vi "frequency measurement(2 notes).vi"() -> (0 "second note":dbl, 3 "first note":dbl)   [LabVIEW 2016]
uses:
  <vilib>/myRIO/Instrument Drivers/Onboard IO/AudioIn Block/typedefs/AudioIn Block Reference.ctl
  <vilib>/myRIO/Common/Instrument Driver Framework/Utilities/typedefs/myRIO Generic Hardware Reference.ctl
  <vilib>/myRIO/Common/Instrument Driver Framework/Utilities/typedefs/Hardware Version Enum.ctl
  <vilib>/myRIO/Common/Instrument Driver Framework/Utilities/typedefs/myRIO v1.0 Reference.ctl
  <vilib>/myRIO/Common/Instrument Driver Framework/Utilities/typedefs/Generic FPGA Reference.ctl
  <vilib>/myRIO/Common/Instrument Driver Framework/myRIO v1.0/AudioIn Block/typedefs/AudioIn Block Channels List.ctl
  <vilib>/myRIO/Common/Instrument Driver Framework/myRIO v1.0/AudioIn Block/typedefs/AudioIn Block Channels Enum.ctl
  <vilib>/myRIO/Common/Instrument Driver Framework/Utilities/typedefs/Analog Scaling Constants.ctl
  <vilib>/userdefined/High Color/nirio_resource_hc.ctl
  <vilib>/myRIO/Common/Instrument Driver Framework/Utilities/vis/Is FPGA Ref Available.vi
  <vilib>/myRIO/Common/Instrument Driver Framework/myRIO v1.0/AudioIn Block/vis/myRIO v1.1 Open Throughput AudioIn (N Samples).vi
  <vilib>/myRIO/Instrument Drivers/Onboard IO/AudioIn Block/vis/Read.vi
  <vilib>/Analysis/2dsp.llb/Real FFT.vi
  <vilib>/myRIO/Common/Instrument Driver Framework/Utilities/vis/Validate Channels.vi
  <vilib>/Utility/VariantDataType/GetNumericInfo.vi
  <vilib>/Utility/error.llb/Error Cluster From Error Code.vi
  <vilib>/myRIO/Common/Instrument Driver Framework/myRIO v1.0/myRIO v1.1 Open Throughput.vi
  <vilib>/myRIO/Common/Instrument Driver Framework/myRIO v1.0/AudioIn Block/vis/myRIO v1.0 Get Scaling Constants AudioIn Block.vi
  <vilib>/myRIO/Common/Instrument Driver Framework/myRIO v1.0/AudioIn Block/vis/myRIO v1.0 Reserve AudioIn Block.vi
  <vilib>/myRIO/Common/Instrument Driver Framework/myRIO v1.0/myRIO v1.0 Close.vi
  <vilib>/myRIO/Common/Instrument Driver Framework/myRIO v1.0/AudioIn Block/vis/myRIO v1.0 AudioIn Block Read.vi
  <vilib>/myRIO/Express VI/Onboard IO/AudioIn/AudioIn Express VI.xnode
  <vilib>/myRIO/Instrument Drivers/Onboard IO/AudioIn Block/vis/myRIO AudioIn N Samples Open.xnode
  <vilib>/Analysis/NI_AALPro.lvlib
  <vilib>/myRIO/Instrument Drivers/Onboard IO/AudioIn Block/AudioIn Block.lvlib
panel:
  out "first record flag":bool
  out "Waveform Graph":dynamicdata(graph)
  out "size(s)":i32
  out "Frequency":dbl
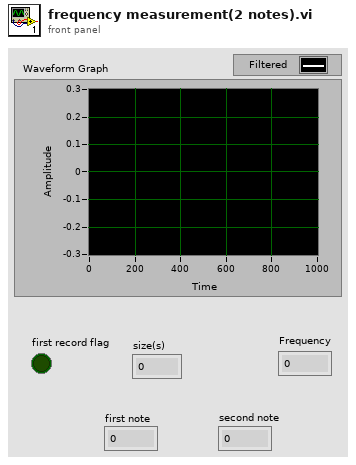
[diagram p1: front panel]
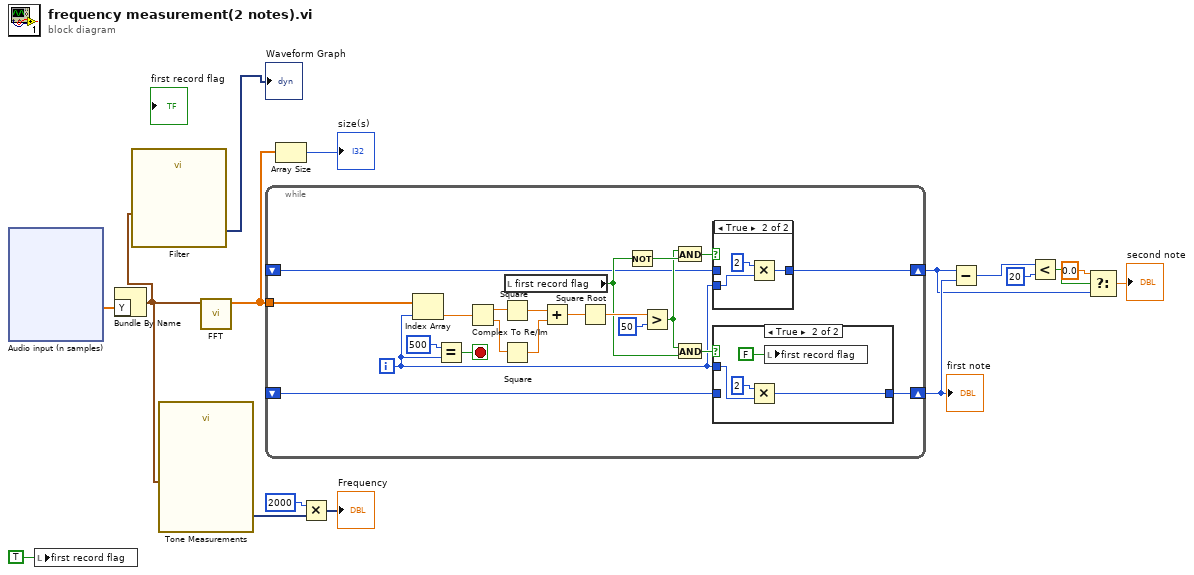
[diagram p0: block diagram]
diagram:
  n1 = xnode "Audio input (n samples)"() -> ("AudioIn/Left (N Samples)"=w12:dbl[])  [unwired: 1 in, 2 out]
  n2 = local write "first record flag"(TRUE) -> ()
  n3 = Bundle By Name("Y"=w12) -> (w3:waveform(dbl))  [unwired: 1 in]
  n4 = call "Filter"("Signal"=w3) -> ("Filtered Signal"=→"Waveform Graph":dynamicdata)  [unwired: 9 in, 1 out]
  n5 = call "Tone Measurements"("Signals"=w3) -> ("Frequency"=w14:dynamicdata)  [unwired: 8 in, 2 out]
  n6 = call-poly <vilib>:"FFT.vi"("X"=w3) -> ("FFT {X}"=w1:cdb[])  [unwired: 9 in, 1 out]
  n7 = while {
    tunnel: w1 -> [w37]
    shift-right: [w26] -> w10
    shift-left: _ -> [w25]
    shift-right: [w18] -> w5
    shift-left: _ -> [w17]
    i -> [w19]
    stop <- w35 stop-if-true
    n8 = Index Array(array=w37, index=w19) -> (element=w34:cdb)
    n9 = Equal?(x=500, y=w19) -> (x = y?=w35:bool)
    n10 = Complex To Re/Im(x + iy=w34) -> (x=w33:dbl, y=w32:dbl)
    n11 = Square(x=w33) -> (x^2=w31:dbl)
    n12 = Square(x=w32) -> (x^2=w30:dbl)
    n13 = local read "first record flag"() -> (w23:bool)
    n14 = Add(x=w31, y=w30) -> (x+y=w29:dbl)
    n15 = Square Root(x=w29) -> (sqrt(x)=w28:dbl)
    n16 = Not(x=w23) -> (.not. x?=w21:bool)
    n17 = Greater?(x=w28, y=50) -> (0:w20:bool)
    n18 = And(x=w20, y=w21) -> (x .and. y?=w22:bool)
    n19 = And(x=w20, y=w23) -> (x .and. y?=w24:bool)
    n20 = case shown="True" w22 {
      tunnel: w19 -> [_ w40]
      tunnel: [w38 w39] -> w18
      tunnel: w17 -> [w38 _]
      frame False {
      }
      frame True {
        n21 = Multiply(x=2, y=w40) -> (x*y=w39:i32)
      }
    }
    n22 = case shown="True" w24 {
      tunnel: w19 -> [_ w45]
      tunnel: [w42 w43] -> w26
      tunnel: w25 -> [w42 _]
      frame False {
      }
      frame True {
        n23 = Multiply(x=2, y=w45) -> (x*y=w43:i32)
        n24 = local write "first record flag"(FALSE) -> ()
      }
    }
  }
  "first note" <- w10
  n25 = Array Size(array=w1) -> (size(s)=→"size(s)":i32)
  n26 = Multiply(x=2000, y=w14) -> (x*y=→"Frequency":dynamicdata)
  n27 = Subtract(x=w5, y=w10) -> (x-y=w9:i32)
  n28 = Less?(x=w9, y=20) -> (x < y?=w7:bool)
  n29 = Select(t=0.0, s=w7, f=w5) -> (s? t:f=→"second note":dbl)
